vi "Volts to Position.vi"(10 "X Voltage":dbl, 11 "X Parameters":T1={"Number of X Steps"=200, "Max X (V)"=2.0, "Min X (V)"=-2.0}) -> (2 "Result":dbl)   [LabVIEW 2011]
uses:
  <vilib>/express/express arith-compare/Formula/XNode/ExpressFormulaBlockNode.xnode
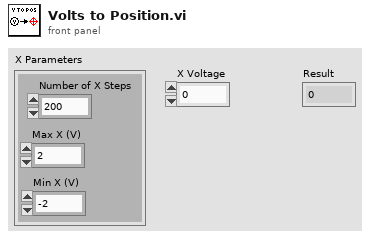
[diagram p1: front panel]
types:
  T1 = cluster{"Number of X Steps":i32, "Max X (V)":dbl, "Min X (V)":dbl}
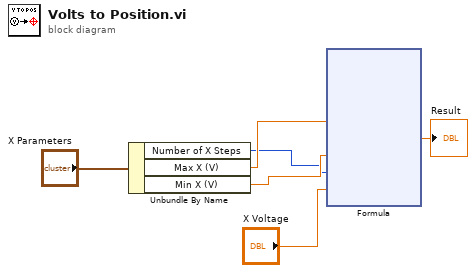
[diagram p0: block diagram]
diagram:
  n1 = Unbundle By Name("X Parameters") -> ("Number of X Steps"=w3:i32, "Max X (V)"=w5:dbl, "Min X (V)"=w4:dbl)
  n2 = xnode "Formula"("X1"=w5, "X2"=w4, "X3"=w3, "X4"="X Voltage") -> ("Result"=→"Result":dbl)  [unwired: 1 in, 1 out]
